vi "get latest state.vi"(11 "t & X":dbl[][](array[numeric])) -> (1 "end element":i32, 2 "Time [s]":dbl, 3 "X_i":dbl[](array[numeric]))   [LabVIEW 2025, in "Dynamic-System.lvclass"]
uses:
  Dynamic-System.lvclass
  Dynamic-System.lvclass/Dynamic-System.ctl
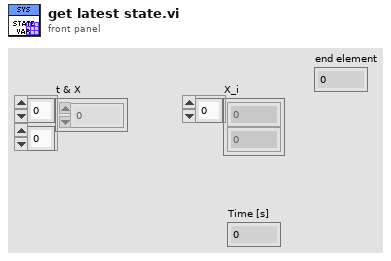
[diagram p1: front panel]
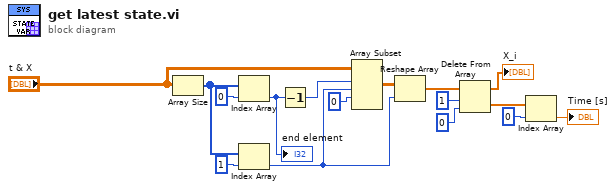
[diagram p0: block diagram]
diagram:
  n1 = Array Size(array="t & X") -> (size(s)=w11:i32[])
  n2 = Index Array(array=w11, index=0) -> (element=w3:i32)
  "end element" <- w3
  n3 = Index Array(array=w11, index=1) -> (element=w1:i32)
  n4 = Decrement(x=w3) -> (x-1=w2:i32)
  n5 = Array Subset(array="t & X", index (row)=w2, length (row)=w1, index (col)=0 ("index")) -> (w13:dbl[][])  [unwired: 1 in]
  n6 = Reshape Array(w13, w1) -> (w14:dbl[])
  n7 = Delete From Array(array=w14, length=1, index=0) -> (deleted portion=w7:dbl[], array with subset deleted=→"X_i":dbl[])
  n8 = Index Array(array=w7, index=0) -> (element=→"Time [s]":dbl)
